vi "Image - BMP string - Image.vi"() -> ()   [LabVIEW 2018]
uses:
  <vilib>/picture/picture.llb/imagedata.ctl
panel:
  in  "File Path":path
  out "Image Out 2":T1(plugin-control)
  out "image data":T2
  out "Image Out":T1(plugin-control)
  in  "Stop (F)":bool
  out "length":i32
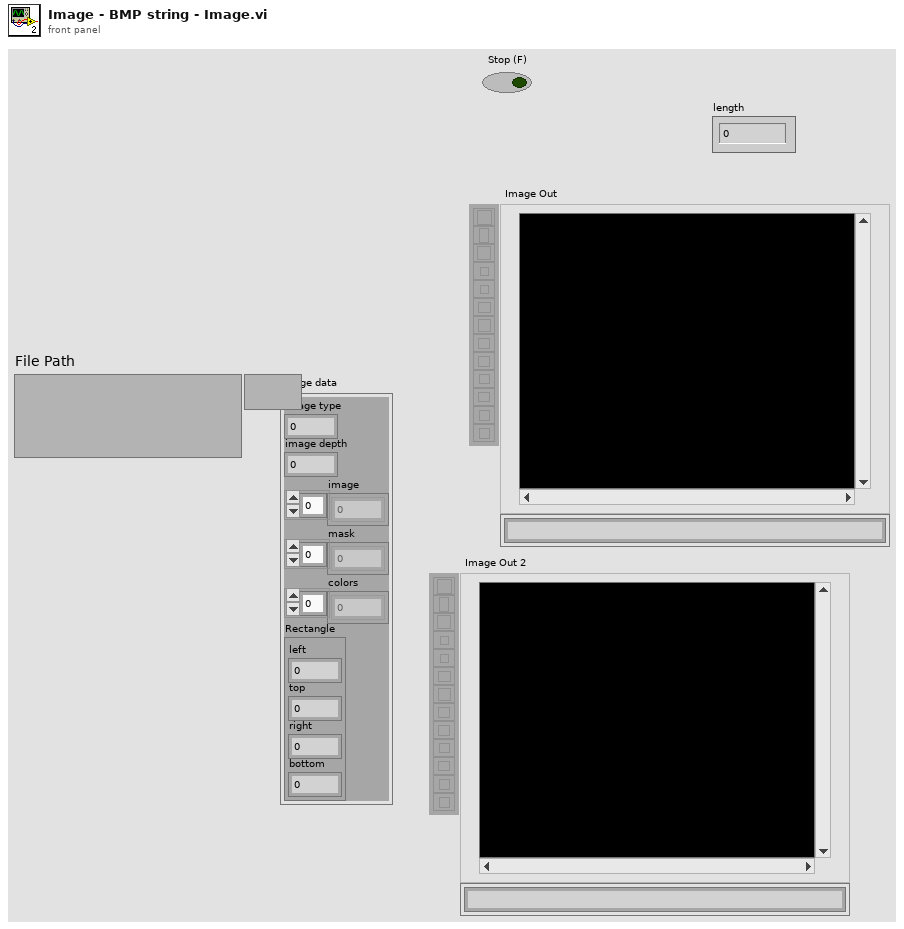
[diagram p1: front panel]
types:
  T1 = typedef "IMAQ Image.ctl" = refnum<image>
  T2 = typedef "imagedata.ctl" = cluster{"image type":i32, "image depth":i32, "image":u8[], "mask":u8[], "colors":u32[], "Rectangle":cluster{"left":i16, "top":i16, "right":i16, "bottom":i16}}
  T3 = typedef "Image Type" = u32
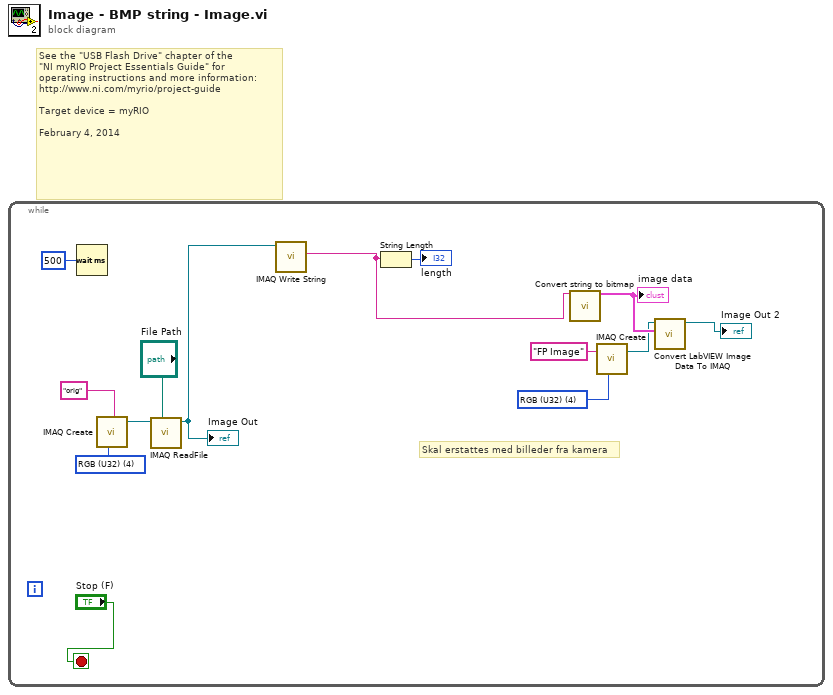
[diagram p0: block diagram]
diagram:
  # "See the \"USB Flash Drive\" chapter of the\n\"NI myRIO Project Essentials Guide\" for\noperating instructions and more information: \nhttp://www.ni.com/myrio/project-guide\n\nTarget device = myRIO\n\nFebruary 4, 2014"
  n1 = while {
    stop <- "Stop (F)" stop-if-true
    w3 = T3 4 items=["Grayscale (U8)", "Grayscale (I16)", "Grayscale (SGL)", "Complex (CSG)", "RGB (U32)", "HSL (U32)", "RGB (U64)"] ("Image Type")
    w9 = T3 4 items=["Grayscale (U8)", "Grayscale (I16)", "Grayscale (SGL)", "Complex (CSG)", "RGB (U32)", "HSL (U32)", "RGB (U64)", "Grayscale (U16)"] ("Image Type")
    # "Skal erstattes med billeder fra kamera"
    n2 = Wait (ms)(milliseconds to wait=u32 500) -> ()  [unwired: 1 out]
    n3 = call "IMAQ Create"("Image Name"="orig", "Image Type"=w3) -> ("New Image"=w5:T1)  [unwired: 2 in, 2 out]
    n4 = call "IMAQ ReadFile"("File Path"="File Path", "Image"=w5) -> ("Image Out"=w1:T1)  [unwired: 3 in, 6 out]
    "Image Out" <- w1
    n5 = call-poly "IMAQ Write String"("Image"=w1) -> ("File String Out"=w12:string)  [unwired: 8 in, 2 out]
    n6 = String Length(string=w12) -> (length=→"length":i32)
    n7 = call "Convert string to bitmap.vi"("data"=w12) -> ("image data"=w11:T2)  [unwired: 13 in, 1 out]
    "image data" <- w11
    n8 = call "IMAQ Create"("Image Name"="FP Image", "Image Type"=w9) -> ("New Image"=w7:T1)  [unwired: 3 in, 1 out]
    n9 = call "Convert LabVIEW Image Data To IMAQ.vi"("Image Data"=w11, "Image In"=w7) -> ("Image Out"=→"Image Out 2":T1)  [unwired: 8 in, 1 out]
  }
